vi "3.vi"() -> ()   [LabVIEW 2015]
panel:
  out "Sample in Queue":u32(slide) scale=0.0..100.0
  out "Queue Loop":dbl(graph)
  out "Loop Rate (ms)":u32
  in  "LoopSpeed":u32(ring) items=["Same as Producer Loop"=50, "Maximum Speed"=0, "2x as Producer"=25, "1/2 as Producer"=100, "1/20 as Producer"=1000]
  out "Loop Rate (ms)":u32
  in  "LoopSpeed":u32(ring) items=["Same as Producer Loop"=50, "Maximum Speed"=0, "2x as Producer"=25, "1/2 as Producer"=100, "1/20 as Producer"=1000]
  out "Missing Sample":i32
  out "Duplicated Sample":i32
  out "Local Variable Loop":dbl(graph)
  in  "Stop Button":bool
  out "Producer Loop":dbl(graph)
  out "Sample":i32
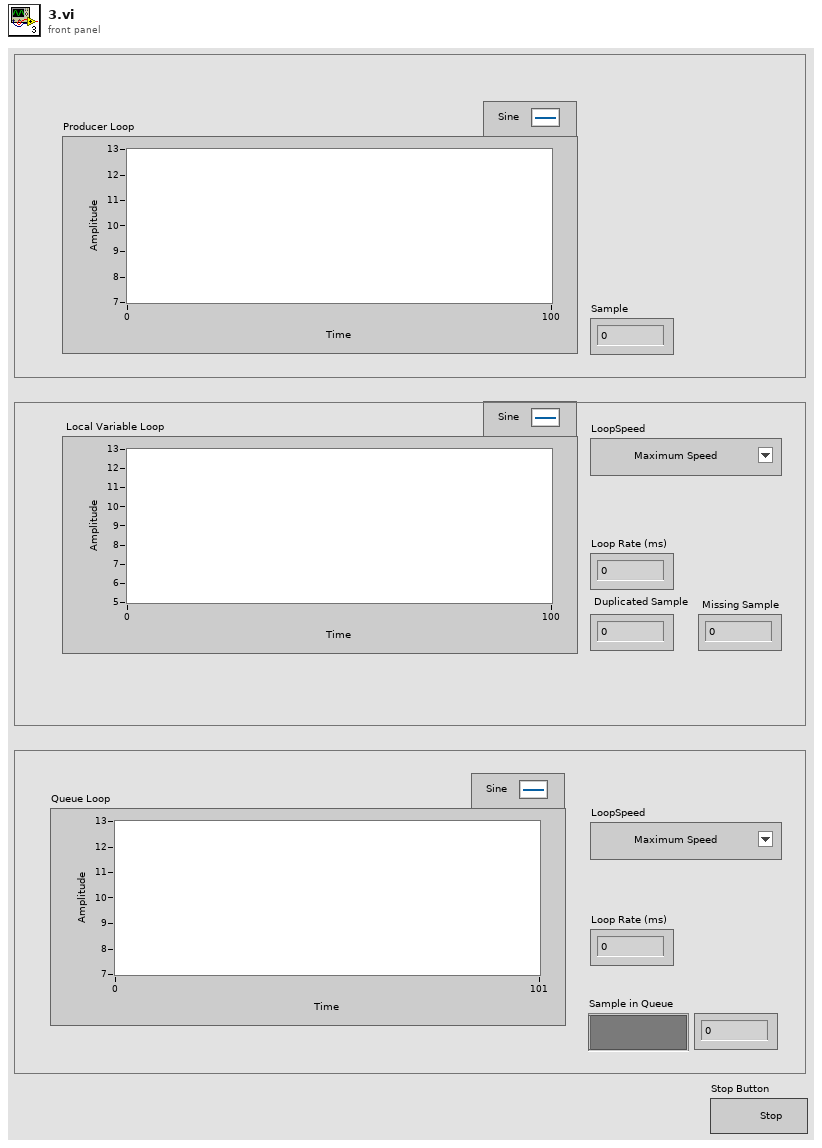
[diagram p1: front panel]
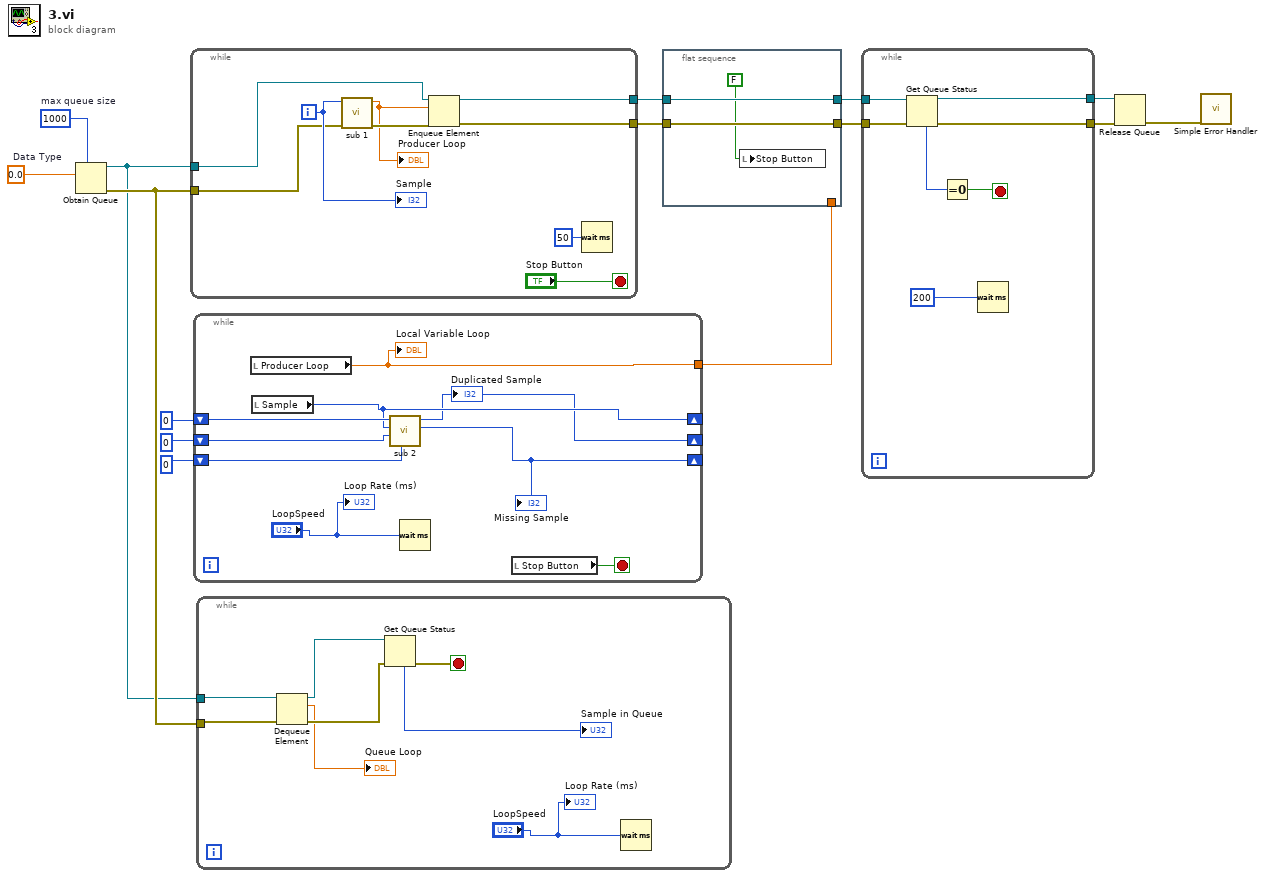
[diagram p0: block diagram]
diagram:
  w14 = 0.0  # Data Type
  w15 = 1000  # max queue size
  n1 = Obtain Queue(max queue size (-1, unlimited)=w15, element data type=w14) -> (queue out=w1:refnum<queue>, error out=w2:errorcluster)  [unwired: 3 in, 1 out]
  n2 = while {
    tunnel: w1 -> [w22]
    tunnel: [w21] -> w11
    tunnel: w2 -> [w20]
    tunnel: [w18] -> w13
    i -> [w24]
    stop <- "Stop Button" stop-if-true
    n3 = call "sub 1.vi"("error in (no error)"=w20, "Numeric"=w24) -> ("error out"=w19:errorcluster, "Sine"=w17:dbl)  [unwired: 8 in]
    "Producer Loop" <- w17
    n4 = Enqueue Element(queue=w22, element=w17, error in (no error)=w19) -> (queue out=w21:refnum<queue>, error out=w18:errorcluster)  [unwired: 1 in, 1 out]
    n5 = Wait (ms)(milliseconds to wait=u32 50) -> ()  [unwired: 1 out]
    "Sample" <- w24
  }
  n6 = while {
    tunnel: [w33] -> w3
    shift-right: [w29] -> _
    shift-left: 0 -> [w30]
    shift-right: [w28] -> _
    shift-left: 0 -> [w31]
    shift-right: [w26] -> _
    shift-left: 0 -> [w32]
    stop <- w27 stop-if-true
    n7 = local read "Producer Loop"() -> (w33:dbl)
    "Local Variable Loop" <- w33
    n8 = local read "Sample"() -> (w29:i32)
    n9 = call "sub 2.vi"("Current Missing Points"=w32, "Previous Producer Iterations"=w31, "Producer Iterations"=w29, "Current Duplicated Points"=w30) -> ("Update Missing Points"=w26:i32, "Updated Duplicated Points"=w28:i32)  [unwired: 6 in]
    "Duplicated Sample" <- w28
    "Missing Sample" <- w26
    n10 = Wait (ms)(milliseconds to wait="LoopSpeed") -> ()  [unwired: 1 out]
    n11 = local read "Stop Button"() -> (w27:bool)
    "Loop Rate (ms)" <- "LoopSpeed"
  }
  n12 = while {
    tunnel: w2 -> [w41]
    tunnel: w1 -> [w40]
    stop <- w37 stop-if-true
    n13 = Dequeue Element(queue=w40, error in (no error)=w41) -> (queue out=w39:refnum<queue>, element=→"Queue Loop":dbl, error out=w38:errorcluster)  [unwired: 1 in, 1 out]
    n14 = Get Queue Status(queue=w39, error in (no error)=w38) -> (error out=w37:errorcluster, # elements in queue=→"Sample in Queue":i32)  [unwired: 1 in, 6 out]
    n15 = Wait (ms)(milliseconds to wait="LoopSpeed") -> ()  [unwired: 1 out]
    "Loop Rate (ms)" <- "LoopSpeed"
  }
  n16 = flat-sequence {
    tunnel: w13 -> [w44]
    tunnel: [w44] -> w12
    tunnel: w11 -> [w43]
    tunnel: [w43] -> w10
    tunnel: w3 -> [_]
    frame #0 {
      n17 = local write "Stop Button"(FALSE) -> ()
    }
  }
  n18 = while {
    tunnel: w12 -> [w49]
    tunnel: w10 -> [w48]
    tunnel: [w46] -> w9
    tunnel: [w45] -> w8
    stop <- w51 stop-if-true
    n19 = Get Queue Status(queue=w48, error in (no error)=w49) -> (queue out=w45:refnum<queue>, error out=w46:errorcluster, # elements in queue=w50:i32)  [unwired: 1 in, 5 out]
    n20 = Equal To 0?(x=w50) -> (x = 0?=w51:bool)
    n21 = Wait (ms)(milliseconds to wait=u32 200 ("millisecond timer value")) -> ()  [unwired: 1 out]
  }
  n22 = Release Queue(queue=w8, error in (no error)=w9) -> (error out=w7:errorcluster)  [unwired: 1 in, 2 out]
  n23 = call <vilib>:"Simple Error Handler.vi"("error in (no error)"=w7) -> ()  [unwired: 4 in, 5 out]
